vi "Parse Log.vi"(7 "Index Timestamp":i64, 9 "Strip Timestamp":bool, 10 "Index Timestamp":string, 11 "Log":string) -> (3 "Filtered Config Entries":string)   [LabVIEW 2021, in "CIFLogs.lvlib"]
uses:
  CIFLogs.lvlib
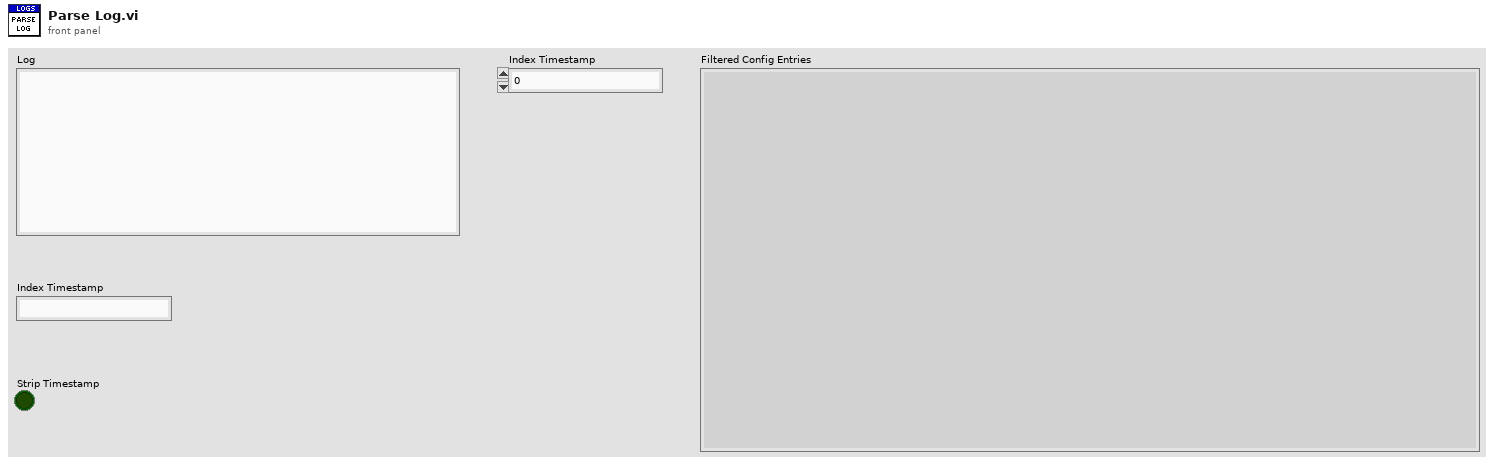
[diagram p1: front panel]
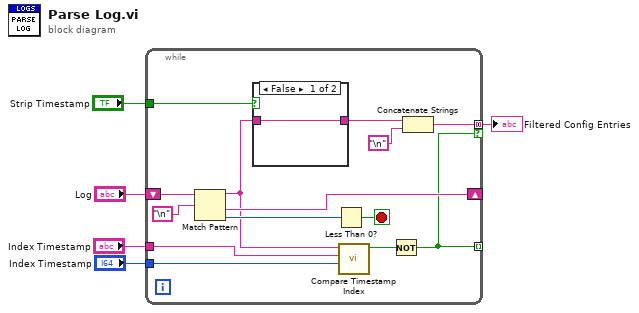
[diagram p0: block diagram]
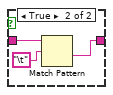
[diagram p2: hidden frame]
diagram:
  n1 = while {
    shift-right: [w18] -> _
    shift-left: "Log" -> [w19]
    tunnel: "Index Timestamp" -> [w9]
    tunnel: [w15] -> w3 mode=concatenating if=w7
    tunnel: "Strip Timestamp" -> [w10]
    tunnel: "Index Timestamp" -> [w8]
    tunnel: [w7] -> _ mode=indexing
    stop <- w6 stop-if-true
    n2 = Match Pattern(string=w19, regular expression="\n") -> (before substring=w14:string, after substring=w18:string, offset past match=w17:i32)  [unwired: 1 in, 1 out]
    n3 = case shown="False" w10 {
      tunnel: w14 -> [w20 w23]
      tunnel: [w20 w22] -> w13
      frame False {
      }
      frame True {
        n4 = Match Pattern(string=w23, regular expression="\t") -> (after substring=w22:string)  [unwired: 1 in, 3 out]
      }
    }
    n5 = Less Than 0?(x=w17) -> (x < 0?=w6:bool)
    n6 = call "Compare Timestamp Index.vi"(9:"Index Timestamp"=w9, 10:"Index Timestamp"=w8, "Log Timestamp"=w14) -> ("Past"=w16:bool)  [unwired: 8 in]
    n7 = Not(x=w16) -> (.not. x?=w7:bool)
    n8 = Concatenate Strings(w13, "\n") -> (w15:string)
  }
  "Filtered Config Entries" <- w3
